vi "Limits(SingleSwitch).vi"(6 "Into Home Limit Is Pos (Motor)":bool, 8 "Power In":dbl format="%#_13g", 11 "Limit Switch Ref":T1={"DevStatus"={"status"=FALSE, "code"=0, "source"=""}, "DIO Channel"=enum."DIO 1", "CntIndex"=enum."Invalid", "Normally Closed"=FALSE}) -> (0 "Power Out":dbl)   [LabVIEW 2018]
uses:
  <vilib>/Rock Robotics/WPI/Switch/WPI_SwitchDevRef.ctl
  <vilib>/Rock Robotics/SystemInterfaces/DIO/FPGA_DIOChannel.ctl
  <vilib>/Rock Robotics/SystemInterfaces/Counter/FPGA_CounterCtrSystemIndex.ctl
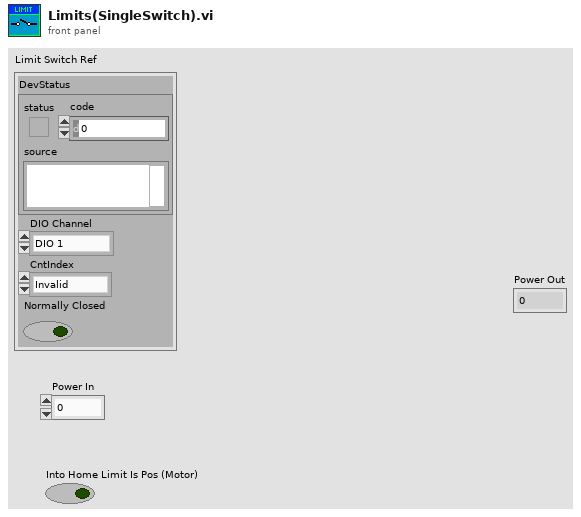
[diagram p1: front panel]
types:
  T1 = typedef "WPI_SwitchDevRef.ctl" = cluster{"DevStatus":errorcluster, "DIO Channel":T2, "CntIndex":T3, "Normally Closed":bool}
  T2 = typedef "FPGA_DIOChannel.ctl" = enum8{"DIO 0", "DIO 1", "DIO 2", "DIO 3", "DIO 4", "DIO 5", "DIO 6", "DIO 7", "DIO 8", "DIO 9", "DIO MXP 0", "DIO MXP 1", "DIO MXP 2", "DIO MXP 3", "DIO MXP 4", "DIO MXP 5", "DIO MXP 6", "DIO MXP 7", "DIO MXP 8", "DIO MXP 9", "DIO MXP 10", "DIO MXP 11", "DIO MXP 12", "DIO MXP 13", "DIO MXP 14", "DIO MXP 15", "SPI Port CS1", "SPI Port CS2", "SPI Port CS3", "SPI Port MISO", "SPI Port MOSI", "Invalid"}
  T3 = typedef "FPGA_CounterCtrSystemIndex.ctl" = enum8{"Ctr 0", "Ctr 1", "Ctr 2", "Ctr 3", "Ctr 4", "Ctr 5", "Ctr 6", "Ctr 7", "Invalid"}
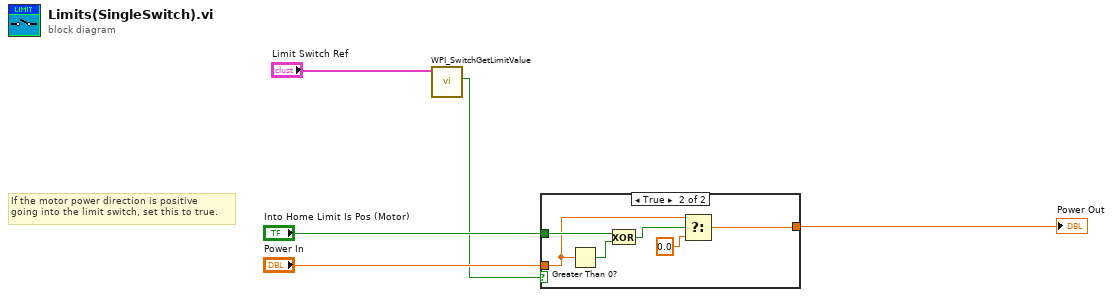
[diagram p0: block diagram]
diagram:
  # "If the motor power direction is positive\ngoing into the limit switch, set this to true."
  n1 = call <vilib>:"WPI_SwitchGetLimitValue.vi"("SwitchDevRef"="Limit Switch Ref") -> ("Switch Pressed"=w1:bool)  [unwired: 8 in, 2 out]
  n2 = case shown="True" w1 {
    tunnel: [w6 w9] -> w4
    tunnel: "Into Home Limit Is Pos (Motor)" -> [_ w8]
    tunnel: "Power In" -> [w6 w7]
    frame False {
    }
    frame True {
      n3 = Greater Than 0?(x=w7) -> (x > 0?=w11:bool)
      n4 = Exclusive Or(1:w11, 2:w8) -> (0:w10:bool)
      n5 = Select(t=w7, s=w10, f=0.0) -> (s? t:f=w9:dbl)
    }
  }
  "Power Out" <- w4
